vi "add photo to GlobalVariables.vi"() -> ()   [LabVIEW 2018]
panel:
  in  "Path":string="C:\\specsheetsConsole\\Documentation\\"
  in  "Name":string="frowny"
  out "new picture":picture
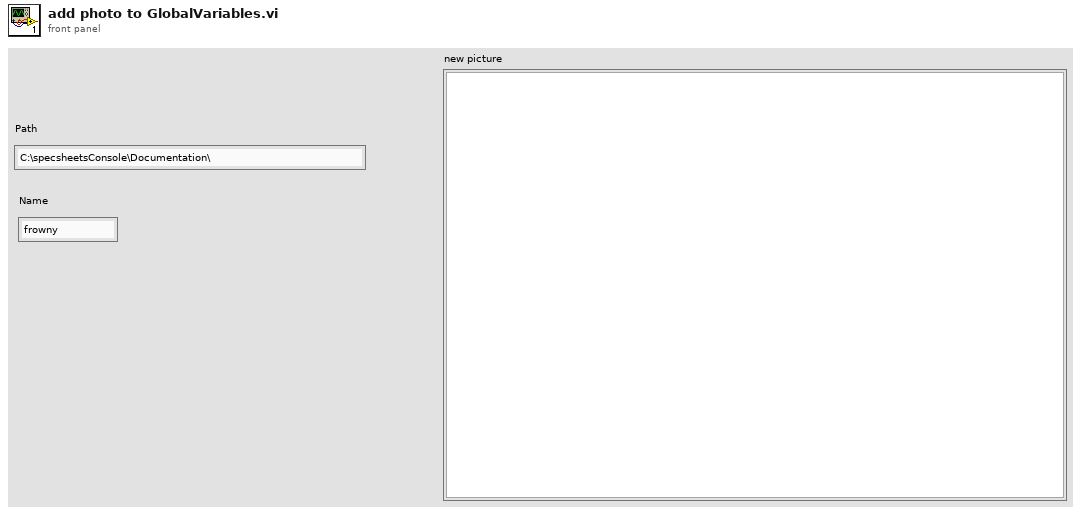
[diagram p1: front panel]
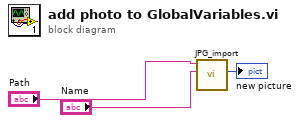
[diagram p0: block diagram]
diagram:
  n1 = call "JPG_import.vi"("File name"="Name", "File path"="Path") -> ("new picture"=→"new picture":picture)  [unwired: 7 in, 2 out]
